vi "calculate height.vi"(8 "Game Parameters":T3={"Upper Limit (m)"=100.0, "Lower Limit (m)"=0.0, "Obstacle time"=20.0, "Obstacle length"=10.0, "fuel decrement"=0.5, "Fuel time"=100.0, "fuel amount"=50.0, "Fuel range"=10, "Death range"=5, "Terrain slope"=35.0, "Speed (km/hr)"=150.0, "Time step (ms)"=30, "Gravity"=-9.81, "Date"="11/03/2016", "High scores path"=path "C:/Users/lz2/Code/LabVIEW/Helicopter/hi scores.txt", "Difficulty"=enum."Normal", "Headstart"=30}, 9 "Thrust (m/s^2)":dbl(slide)=21.212121212121215 scale=0.0..50.0, 10 "Thrusters on?":bool, 11 "Arrays and Heights":T1={"Score Array"=[], "Lowest high score"=0.0, "Score"=0.0, "Ceiling"=0.0, "Floor"=0.0, "Ceiling Array"=[], "Floor array"=[], "Helicopter height"=0.0, "Helicopter array"=[], "Fuel"=300.0, "Fuel array"=[], "fuel counter"=0, "obstacle counter"=0, "Obstacle array"=[], "helicopter v_0"=0.0, "helicopter a_0"=0.0, "Obstacle height"=300.0}) -> (1 "Acceleration (m/s^2)":dbl(knob)=-7.385757575757571 scale=-10.0..10.0, 2 "Decrement fuel?":bool, 3 "Arrays and Heights":T1={"Score Array"=[], "Lowest high score"=0.0, "Score"=0.0, "Ceiling"=0.0, "Floor"=0.0, "Ceiling Array"=[], "Floor array"=[], "Helicopter height"=0.0, "Helicopter array"=[], "Fuel"=300.0, "Fuel array"=[], "fuel counter"=0, "obstacle counter"=0, "Obstacle array"=[], "helicopter v_0"=0.0, "helicopter a_0"=0.0, "Obstacle height"=300.0})   [LabVIEW 2017]
uses:
  controls/arrays and heights.ctl
  controls/scores.ctl
  controls/game parameters.ctl
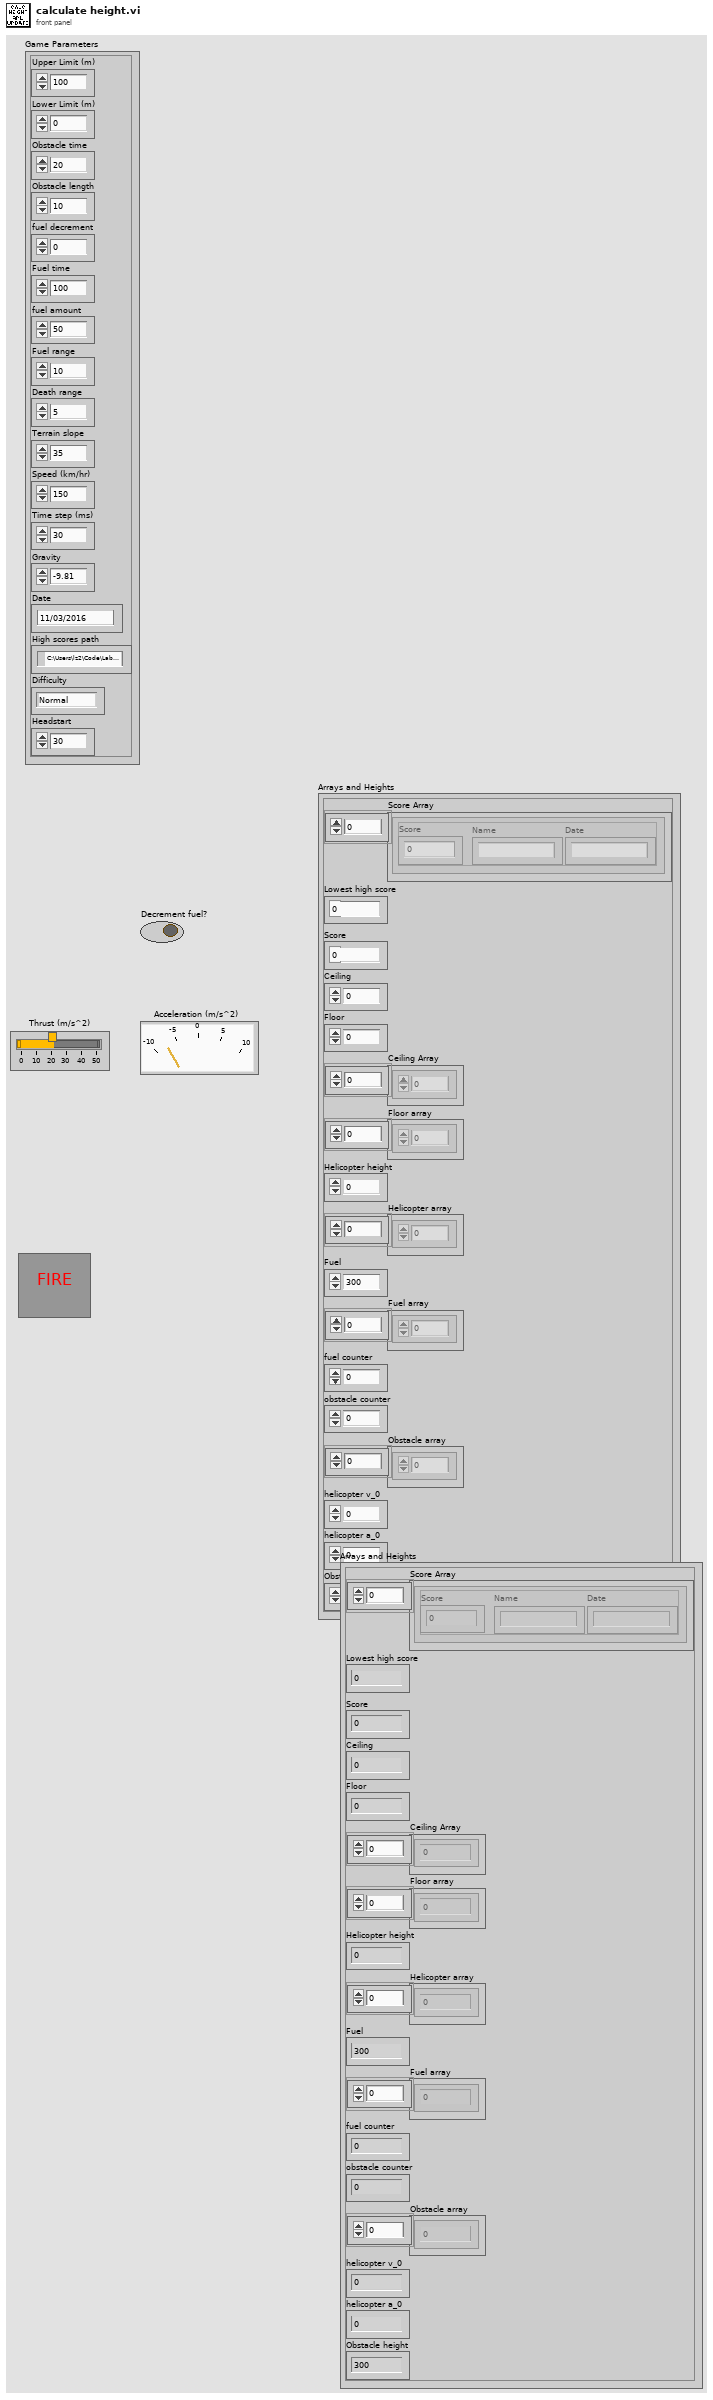
[diagram p1: front panel]
types:
  T1 = typedef "arrays and heights.ctl" = cluster{"Score Array":T2[], "Lowest high score":dbl, "Score":dbl, "Ceiling":dbl, "Floor":dbl, "Ceiling Array":dbl[], "Floor array":dbl[], "Helicopter height":dbl, "Helicopter array":dbl[], "Fuel":dbl, "Fuel array":dbl[], "fuel counter":i32, "obstacle counter":i32, "Obstacle array":dbl[], "helicopter v_0":dbl, "helicopter a_0":dbl, "Obstacle height":dbl}
  T2 = typedef "scores.ctl" = cluster{"Score":dbl, "Name":string, "Date":string}
  T3 = typedef "game parameters.ctl" = cluster{"Upper Limit (m)":dbl, "Lower Limit (m)":dbl, "Obstacle time":dbl, "Obstacle length":dbl, "fuel decrement":dbl, "Fuel time":dbl, "fuel amount":dbl, "Fuel range":i32, "Death range":i32, "Terrain slope":dbl, "Speed (km/hr)":dbl, "Time step (ms)":u32, "Gravity":dbl, "Date":string, "High scores path":path, "Difficulty":enum16{"Easy", "Normal", "Hard"}, "Headstart":u32}
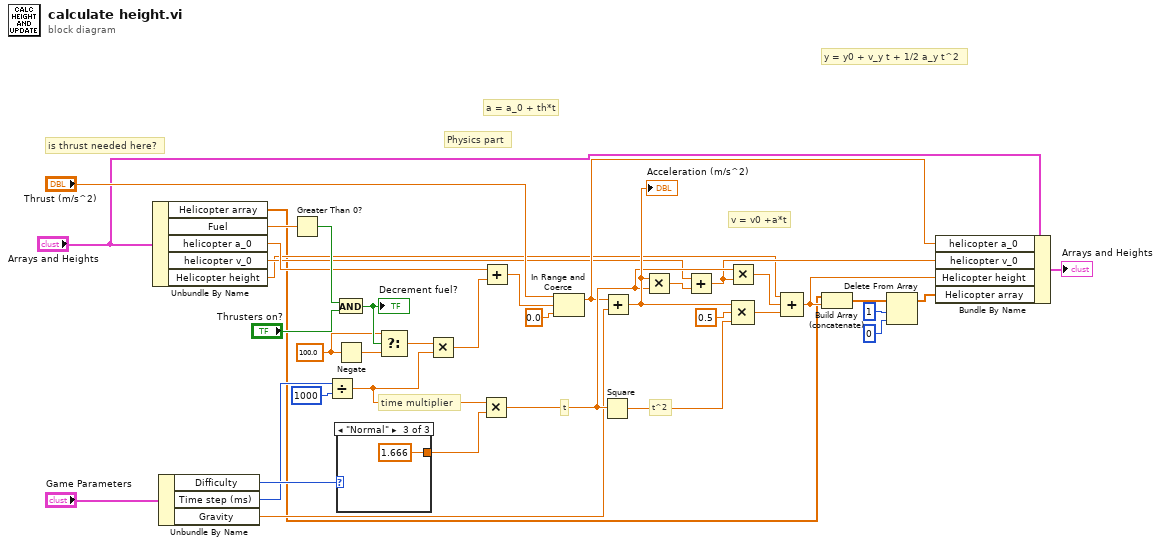
[diagram p0: block diagram]
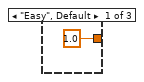
[diagram p2: hidden frame]
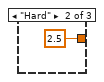
[diagram p3: hidden frame]
diagram:
  w29 = 100.0 ("Jerk (m/s^3)")
  # "time multiplier"
  # "is thrust needed here?"
  # "a = a_0 + th*t"
  # "v = v0 +a*t"
  # "Physics part"
  # "t"
  # "y = y0 + v_y t + 1/2 a_y t^2"
  # "t^2"
  n1 = Unbundle By Name("Arrays and Heights") -> ("Helicopter array"=w2:dbl[], "Fuel"=w18:dbl, "helicopter a_0"=w14:dbl, "helicopter v_0"=w9:dbl, "Helicopter height"=w7:dbl)
  n2 = Unbundle By Name("Game Parameters") -> ("Difficulty"=w16:enum16{"Easy", "Normal", "Hard"}, "Time step (ms)"=w15:u32, "Gravity"=w8:dbl)
  n3 = Greater Than 0?(x=w18) -> (x > 0?=w36:bool)
  n4 = Divide(x=w15, y=u32 1000) -> (x/y=w19:dbl)
  n5 = And(x=w36, y="Thrusters on?") -> (x .and. y?=w37:bool)
  "Decrement fuel?" <- w37
  n6 = Negate(x=w29) -> (-x=w30:dbl)
  n7 = case shown="\"Normal\"" w16 {
    tunnel: [1.0 ("y") 2.5 ("y") 1.666 ("y")] -> w34
    frame "Easy", Default {
    }
    frame "Hard" {
    }
    frame "Normal" {
    }
  }
  n8 = Select(t=w29, s=w37, f=w30) -> (s? t:f=w31:dbl)
  n9 = Multiply(x=w31, y=w19) -> (x*y=w27:dbl)
  n10 = Multiply(x=w19, y=w34) -> (x*y=w20:dbl)
  n11 = Add(x=w14, y=w27) -> (x+y=w28:dbl)
  n12 = In Range and Coerce(upper limit="Thrust (m/s^2)", x=w28, lower limit=0.0) -> (coerced(x)=w11:dbl)  [unwired: 1 out]
  n13 = Square(x=w20) -> (x^2=w24:dbl)
  n14 = Add(x=w11, y=w8) -> (x+y=w21:dbl)
  "Acceleration (m/s^2)" <- w21
  n15 = Multiply(x=w21, y=w20) -> (x*y=w25:dbl)
  n16 = Add(x=w9, y=w25) -> (x+y=w10:dbl)
  n17 = Multiply(x=w20, y=w10) -> (x*y=w26:dbl)
  n18 = Compound Arithmetic op=MULTIPLY(w21, 0.5 ("value"), w24) -> (w33:dbl)
  n19 = Compound Arithmetic op=ADD(w7, w26, w33) -> (w3:dbl)
  n20 = Build Array (concatenate)(w2, w3) -> (w6:dbl[])
  n21 = Delete From Array(array=w6, length=1, index=0) -> (array with subset deleted=w1:dbl[])  [unwired: 1 out]
  n22 = Bundle By Name(cluster="Arrays and Heights", "helicopter a_0"=w11, "helicopter v_0"=w10, "Helicopter height"=w3, "Helicopter array"=w1) -> (→"Arrays and Heights":T1)
